vi "RSZVB Set Fixture Compensation Direct Compensation.vi"(8 "error in (no error)":errorcluster {"code" format="%.0x"}, 10 "Direct Compensation (On)":bool=TRUE, 11 "VISA session":refnum<visa-resource-name>) -> (0 "error out":errorcluster {"code" format="%.0x"}, 3 "dup VISA session":refnum<visa-resource-name>)   [LabVIEW 2011]
doc: "This VI configures direct compensation.\n\nRemote-control command(s):\n[SENSe<Ch>:]CORRection:COLLect:FIXTure:LMParameter[:STATe]"
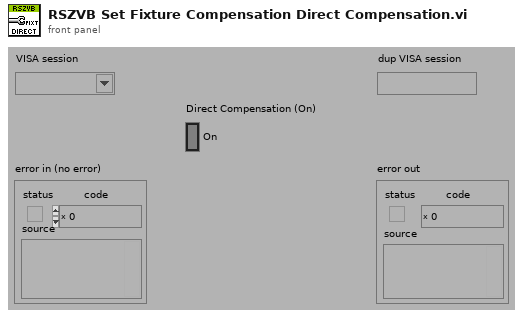
[diagram p1: front panel]
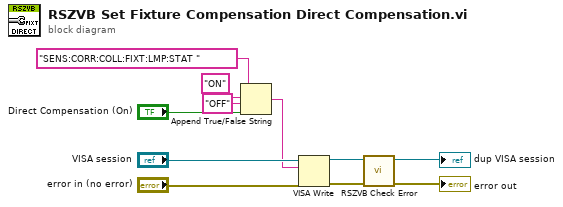
[diagram p0: block diagram]
diagram:
  n1 = Append True/False String(1:"Direct Compensation (On)", 2:"OFF" ("false string"), 3:"ON" ("true string"), 4:"SENS:CORR:COLL:FIXT:LMP:STAT " ("string (\"\")")) -> (0:w5:string)
  n2 = VISA Write(VISA resource name="VISA session", write buffer=w5, error in (no error)="error in (no error)") -> (VISA resource name out=w3:refnum<visa-resource-name>, error out=w4:errorcluster)  [unwired: 1 out]
  n3 = call "RSZVB Check Error.vi"("error in (no error)"=w4, "VISA session"=w3) -> ("error out"=→"error out":errorcluster, "dup VISA session"=→"dup VISA session":refnum<visa-resource-name>)  [unwired: 8 in]
